vi "FTW-Actor-HandleError.vi"(0 "FTW Actor Instance":refnum<class "FTW-ActorInstance.lvclass">, 5 "Explanation":string, 11 "error in":errorcluster) -> (4 "FTW Actor Instance out":refnum<class "FTW-ActorInstance.lvclass">, 6 "Exception occured?":T1, 8 "Serialized Event":string, 15 "error out":errorcluster)   [LabVIEW 2015, in "FTW-ActorInstance.lvclass"]
uses:
  FTW-ActorInstance.lvclass
  Error/FTW-ERR-ExceptionType.ctl
  FTW-ActorInstance.lvclass/FTW-ActorInstance.ctl
panel:
  # "Inputs"
  # "Outputs"
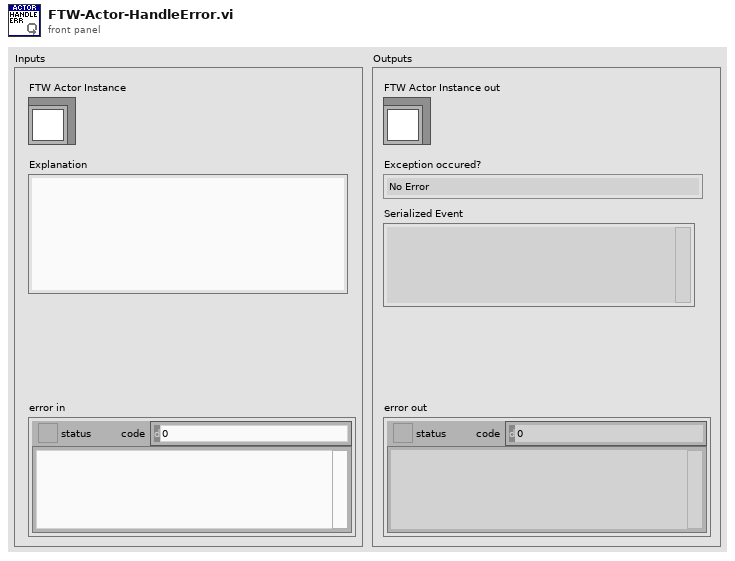
[diagram p1: front panel]
types:
  T1 = typedef "FTW-ERR-ExceptionType.ctl" = enum16{"No Error", "Error", "Warning"}
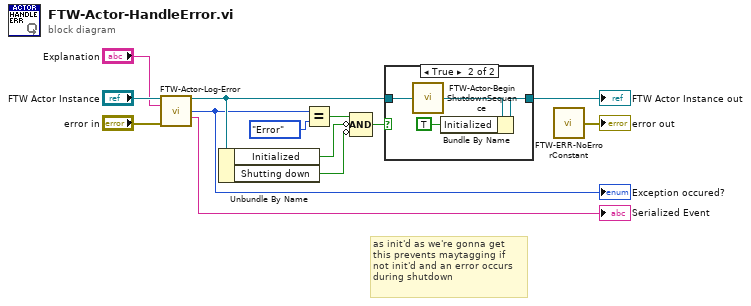
[diagram p0: block diagram]
diagram:
  # "as init'd as we're gonna get\nthis prevents maytagging if\nnot init'd and an error occurs\nduring shutdown"
  n1 = call-dynamic "FTW-Actor-Log-Error.vi"("FTW Actor Instance"="FTW Actor Instance", "Explanation"="Explanation", "Error to Log"="error in") -> ("FTW Actor Instance out"=w4:refnum<class "FTW-ActorInstance.lvclass">, "Exception"=w3:T1, "Serialized Event"=→"Serialized Event":string)  [unwired: 9 in, 1 out]
  "Exception occured?" <- w3
  n2 = Unbundle By Name(w4) -> ("Initialized"=w7:bool, "Shutting down"=w1:bool)
  n3 = Equal?(x=w3, y=FTW-ERR-ExceptionType."Error") -> (x = y?=w6:bool)
  n4 = Compound Arithmetic op=AND(w6, invert w7, invert w1) -> (w5:bool)
  n5 = case shown="True" w5 {
    tunnel: w4 -> [w14 w18]
    tunnel: [w14 w16] -> w2
    frame False {
    }
    frame True {
      n6 = call "FTW-Actor-BeginShutdownSequence.vi"("FTW Actor Instance"=w18) -> ("FTW Actor Instance out"=w17:refnum<class "FTW-ActorInstance.lvclass">)  [unwired: 3 in]
      n7 = Bundle By Name(cluster=w17, "Initialized"=TRUE) -> (w16:refnum<class "FTW-ActorInstance.lvclass">)
    }
  }
  "FTW Actor Instance out" <- w2
  n8 = call "FTW-ERR-NoErrorConstant.vi"() -> ("no error"=→"error out":errorcluster)
